vi "Measurement Logic.vi"() -> ()   [LabVIEW 2021, in "Single Tone_DAC.lvlib"]
uses:
  Single Tone_DAC.lvlib
  Measurement Configuration.ctl
  Measurement Results.ctl
  <vilib>/MeasurementLink/MeasurementLink Measurement Server/Measure Call Context/Measure Call Context.lvclass
  <instrlib>/niScope/Acquire/Fetch/niScope Multi Fetch WDT.vi
panel:
  out "measure call context out":refnum<class "Measure Call Context.lvclass">
  in  "measure call context in":refnum<class "Measure Call Context.lvclass">
  out "measurement results":T1 {"ENOB" format="%_6g"; "THD (dB)" format="%_6g"; "SINAD (dB)" format="%_6g"; "SNR (dB)" format="%_6g"; "SFDR (dBc)" format="%_6g"; "Amplitude (dB)" format="%_6g"; "Amplitude (V)" format="%_6g"; "Frequency (Hz)" format="%_6g"; "dt" format="%_6g"; "Frequency domain" format="%_6g"; "Time domain" format="%_6g"}
  in  "measurement configuration":T2={"Digital resource"="", "DAC channel"=0, "Number of bits"=32, "Full scale range (V)"=3968.0, "Frequency (Hz)"=5.0, "Amplitude start (V)"=5.5, "Amplitude stop (V)"=5.5, "Number of cycles"=10, "Scope resource"="", "Scope channel"="", "Scope sample rate (Hz)"=1000000.0, "Scope samples"=1000000, "Scope range (V)"=10.0} {"Scope sample rate (Hz)" format="%#_6p"}
  out "error out":errorcluster
  in  "error in":errorcluster
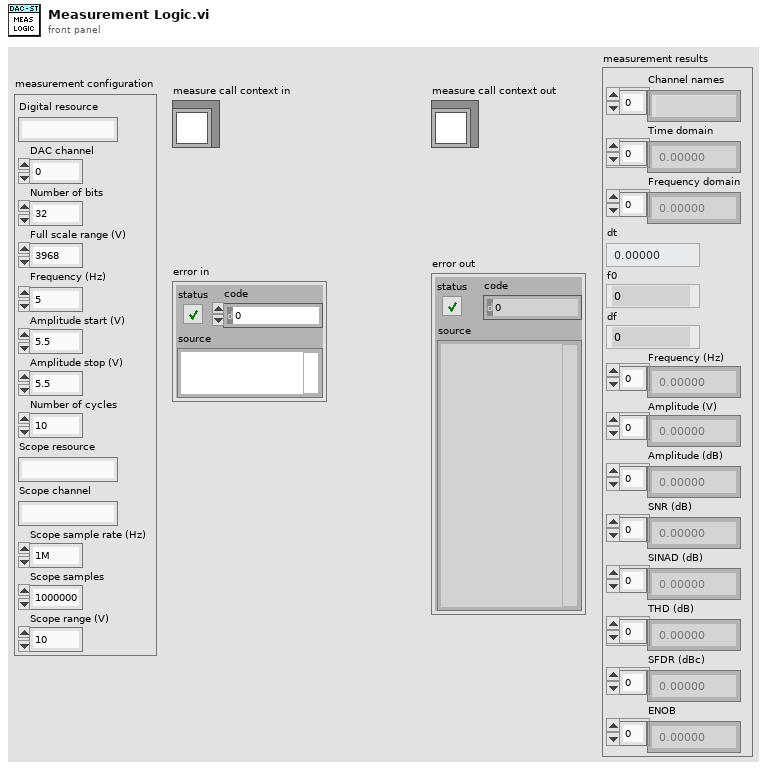
[diagram p1: front panel]
types:
  T1 = typedef "Single Tone_DAC.lvlib/Measurement Results.ctl" = cluster{"Channel names":string[], "Time domain":dbl[], "Frequency domain":dbl[], "dt":dbl, "f0":dbl, "df":dbl, "Frequency (Hz)":dbl[], "Amplitude (V)":dbl[], "Amplitude (dB)":dbl[], "SNR (dB)":dbl[], "SINAD (dB)":dbl[], "THD (dB)":dbl[], "SFDR (dBc)":dbl[], "ENOB":dbl[]}
  T2 = typedef "Single Tone_DAC.lvlib/Measurement Configuration.ctl" = cluster{"Digital resource":string, "DAC channel":u32, "Number of bits":u32, "Full scale range (V)":dbl, "Frequency (Hz)":dbl, "Amplitude start (V)":dbl, "Amplitude stop (V)":dbl, "Number of cycles":u32, "Scope resource":string, "Scope channel":string, "Scope sample rate (Hz)":dbl, "Scope samples":u32, "Scope range (V)":dbl}
  T3 = cluster{"Detected Frequency (Hz)":dbl, "Detected Amplitude (Vpk-pk)":dbl, "SNR (dB)":dbl, "THD (dB)":dbl, "SINAD (dB)":dbl, "SFDR (dBC)":dbl, "ENOB":dbl}
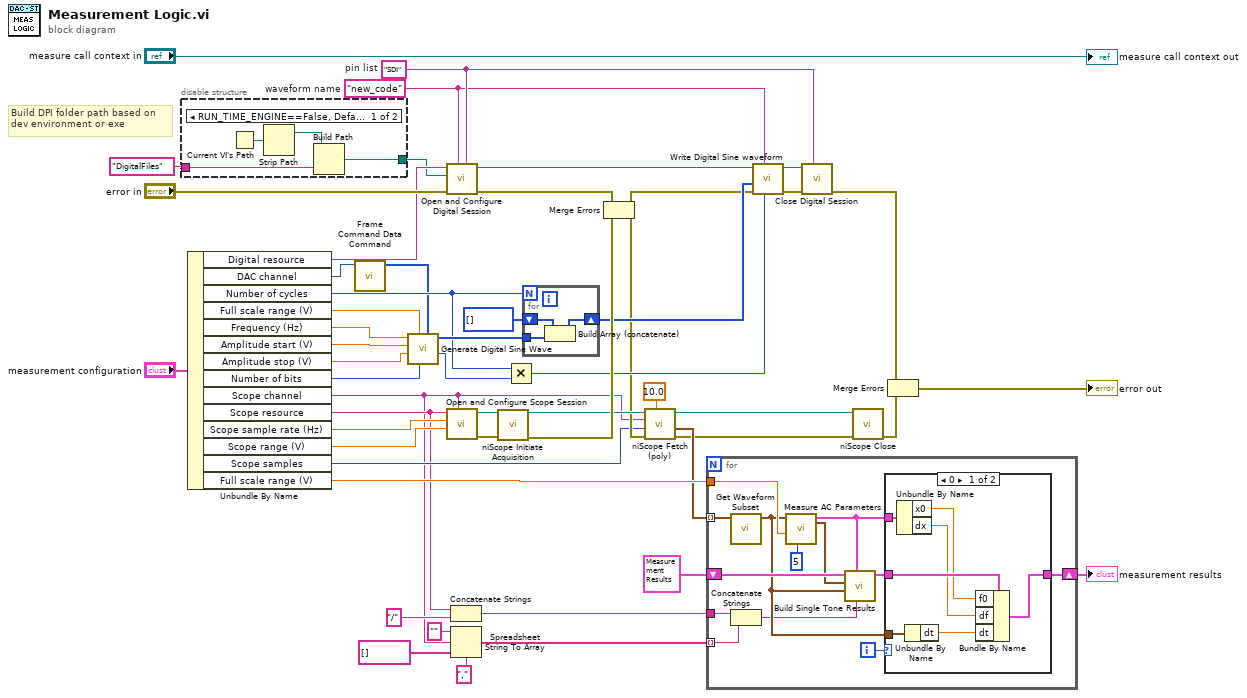
[diagram p0: block diagram]
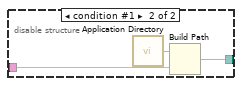
[diagram p3: hidden frame]
diagram:
  w49 = "SDI"  # pin list
  w29 = "new_code"  # waveform name
  # "Build DPI folder path based on\ndev environment or exe"
  n1 = disable-structure shown="RUN_TIME_ENGINE==False, Default" {
    disable-tunnel: "DigitalFiles" -> [w53 w57]
    disable-tunnel: [w52 w56] -> w44
    frame condition #0 (active) {
      n2 = Current VI's Path() -> (path=w55:path)
      n3 = Strip Path(path=w55) -> (stripped path=w54:path)  [unwired: 1 out]
      n4 = Build Path(base path=w54, name or relative path=w53) -> (appended path=w52:path)
    }
    frame condition #1 {
      n5 = call <vilib>:"Application Directory.vi"() -> ("Application Directory"=w58:path)
      n6 = Build Path(base path=w58, name or relative path=w57) -> (appended path=w56:path)
    }
  }
  n7 = Unbundle By Name("measurement configuration") -> ("Digital resource"=w50:string, "DAC channel"=w7:u32, "Number of cycles"=w11:u32, "Full scale range (V)"=w20:dbl, "Frequency (Hz)"=w18:dbl, "Amplitude start (V)"=w17:dbl, "Amplitude stop (V)"=w16:dbl, "Number of bits"=w19:u32, "Scope channel"=w5:string, "Scope resource"=w14:string, "Scope sample rate (Hz)"=w42:dbl, "Scope range (V)"=w41:dbl, "Scope samples"=w25:u32, "Full scale range (V)"=w24:dbl)
  n8 = call "Frame Command Data Command.vi"("DAC channel"=w7) -> ("Command_Data array"=w6:i16[])  [unwired: 10 in]
  n9 = call "Generate Digital Sine Wave.vi"("Command_Data array"=w6, "Number of Bits"=w19, "Full scale range"=w20, "Amplitude stop"=w16, "Amplitude start"=w17, "Frequency"=w18) -> ("Points per cycle"=w10:i32, "Digital Sine waveform"=w35:i16[])  [unwired: 4 in]
  n10 = call "Open and Configure Digital Session.vi"("pin list"=w49, "waveform name"=w29, "error in"="error in", "Digital pattern folder"=w44, "Digital resource"=w50) -> ("error out"=w36:errorcluster, "Digital session"=w33:refnum<k15>)  [unwired: 5 in]
  n11 = call "Open and Configure Scope Session.vi"("Channels"=w5, "Vertical range"=w41, "Sample rate"=w42, "Scope resource"=w14) -> ("error out"=w39:errorcluster, "Scope seesion out"=w40:refnum<k15>)  [unwired: 6 in]
  n12 = Concatenate Strings(w14, "/" ("string")) -> (w12:string)
  n13 = Spreadsheet String To Array(delimiter (Tab)=",", format string="", spreadsheet string=w5, array type (2D Dbl)=string[] []) -> (array=w1:string[])
  n14 = call <instrlib>:"niScope Initiate Acquisition.vi"("instrument handle"=w40, "error in"=w39) -> ("instrument handle out"=w27:refnum<k15>, "error out"=w37:errorcluster)  [unwired: 12 in]
  n15 = Multiply(x=w11, y=w10) -> (x*y=w30:u32)
  n16 = for {
    N: w11 -> [_]
    tunnel: w35 -> [w61]
    shift-right: [w60] -> w34
    shift-left: i16[] [] -> [w59]
    n17 = Build Array (concatenate)(w59, w61) -> (w60:i16[])
  }
  n18 = Merge Errors(w36, w37) -> (w26:errorcluster)
  n19 = call-poly <instrlib>:"niScope Fetch (poly).vi"("timeout"=10.0, "error in"=w26, "numSamples"=w25, "channels"=w5, "instrument handle"=w27) -> ("error out"=w15:errorcluster, "wfm"=w23:waveform(dbl)[], "instrument handle out"=w22:refnum<k15>)  [unwired: 3 in, 1 out]
  n20 = for {
    tunnel: w24 -> [w74]
    tunnel: w23 -> [w73] mode=indexing
    tunnel: w12 -> [w64]
    shift-right: [w65] -> w8
    shift-left: T1 {"Channel names"=[], "Time domain"=[], "Frequency domain"=[], "dt"=0.0, "f0"=0.0, "df"=0.0, "Frequency (Hz)"=[], "Amplitude (V)"=[], "Amplitude (dB)"=[], "SNR (dB)"=[], "SINAD (dB)"=[], "THD (dB)"=[], "SFDR (dBc)"=[], "ENOB"=[]} ("measurement results") -> [w71]
    tunnel: w1 -> [w63] mode=indexing
    i -> [w69]
    n21 = call "Get Waveform Subset.vi"("wfm in"=w73) -> ("wfm out"=w67:waveform(dbl))  [unwired: 10 in]
    n22 = Concatenate Strings(w64, w63) -> (w62:string)
    n23 = call "Measure AC Parameters.vi"("maximum harmonic"=5, "Full scale range"=w74, "Acquired waveform"=w67) -> ("Single tone results"=w70:T3, "FFT"=w66:cluster{"x0":dbl, "dx":dbl, "magnitude":dbl[]})  [unwired: 6 in, 1 out]
    n24 = call "Build Single Tone Results.vi"("Channel name"=w62, "FFT"=w66, "Time domain"=w67, "Single tone results"=w70, "Meas Results In"=w71) -> ("Meas Results Out"=w68:T1)  [unwired: 6 in]
    n25 = case shown="0" w69 {
      tunnel: w68 -> [w81 w82]
      tunnel: w67 -> [w80 _]
      tunnel: w66 -> [w78 _]
      tunnel: [w75 w82] -> w65
      frame 0 {
        n26 = Unbundle By Name(w78) -> ("x0"=w76:dbl, "dx"=w77:dbl)
        n27 = Unbundle By Name(w80) -> ("dt"=w79:dbl)
        n28 = Bundle By Name(cluster=w81, "f0"=w76, "df"=w77, "dt"=w79) -> (w75:T1)
      }
      frame 1, Default {
      }
    }
  }
  "measurement results" <- w8
  n29 = call "Write Digital Sine waveform.vi"("reg0 value"=w30, "Waveform name"=w29, "error in"=w26, "Waveform data"=w34, "Digital session"=w33) -> ("error out"=w31:errorcluster, "Digital session out"=w32:refnum<k15>)  [unwired: 5 in]
  n30 = call "Close Digital Session.vi"("pin list"=w49, "error in"=w31, "Digital session"=w32) -> ("error out"=w48:errorcluster)  [unwired: 8 in]
  n31 = call <instrlib>:"niScope Close.vi"("instrument handle"=w22, "error in"=w15) -> ("error out"=w21:errorcluster)  [unwired: 13 in]
  n32 = Merge Errors(w48, w21) -> (→"error out":errorcluster)
  "measure call context out" <- "measure call context in"
